vi "Start Acquisition.vi"(8 "error in (no error)":errorcluster, 11 "Acquisition in":refnum<class "Acquisition.lvclass">) -> (0 "error out":errorcluster, 3 "Acquisition out":refnum<class "Acquisition.lvclass">)   [LabVIEW 2018, in "Acquisition.lvlib" / "Acquisition.lvclass"]
uses:
  Acquisition.lvclass
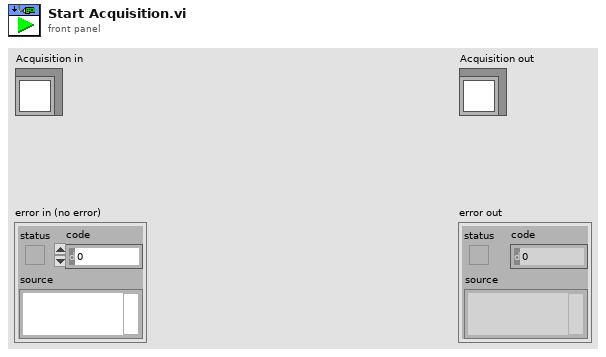
[diagram p1: front panel]
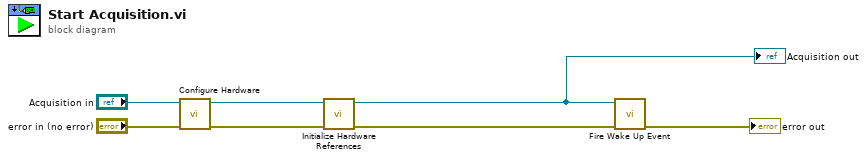
[diagram p0: block diagram]
diagram:
  n1 = call-dynamic "Configure Hardware.vi"("error in (no error)"="error in (no error)", "Acquisition in"="Acquisition in") -> ("error out"=w5:errorcluster, "Acquisition out"=w4:refnum<class "Acquisition.lvclass">)  [unwired: 8 in]
  n2 = call-dynamic "Initialize Hardware References.vi"("error in (no error)"=w5, "Acquisition in"=w4) -> ("error out"=w2:errorcluster, "Acquisition out"=w3:refnum<class "Acquisition.lvclass">)  [unwired: 8 in]
  "Acquisition out" <- w3
  n3 = call "Fire Wake Up Event.vi"("error in (no error)"=w2, "Acquisition in"=w3) -> ("error out"=→"error out":errorcluster)  [unwired: 9 in]
